vi "template (reverse).vi"() -> ()   [LabVIEW 2012]
uses:
  <vilib>/Analysis/1siggen.llb/Ramp Pattern by Samples.vi
  <vilib>/Analysis/NI_AALBase.lvlib
panel:
  out "Sorted Array":variant[](array[variant])
  out "Sorted Keys":dbl[](array[numeric])
  in  "Keys":dbl[](array[numeric])
  in  "Array":variant[](array[variant])
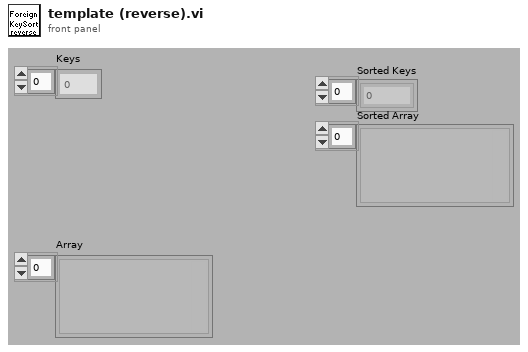
[diagram p1: front panel]
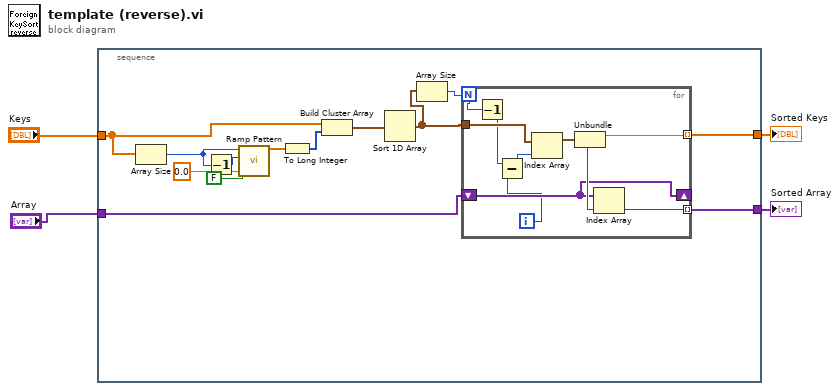
[diagram p0: block diagram]
diagram:
  n1 = stacked-sequence {
    tunnel: "Keys" -> [w11]
    tunnel: "Array" -> [w9]
    tunnel: [w8] -> w2
    tunnel: [w7] -> w1
    frame #0 {
      n2 = Array Size(array=w11) -> (size(s)=w16:i32)
      n3 = Decrement(x=w16) -> (x-1=w17:i32)
      n4 = call-poly <vilib>:"Ramp Pattern.vi"("exclude end?"=FALSE, "start"=0.0, "end"=w17, "samples"=w16) -> ("Ramp Pattern"=w13:dbl[])  [unwired: 6 in, 1 out]
      n5 = To Long Integer(number=w13) -> (32bit integer=w12:i32[])
      n6 = Build Cluster Array(w11, w12) -> (w10:cluster{"Numeric":dbl, i32}[])
      n7 = Sort 1D Array(array=w10) -> (sorted array=w6:cluster{"Numeric":dbl, i32}[])
      n8 = Array Size(array=w6) -> (size(s)=w5:i32)
      n9 = for {
        N: w5 -> [w19]
        tunnel: w6 -> [w27]
        shift-right: [w24] -> _
        shift-left: w9 -> [w24]
        tunnel: [w25] -> w8 mode=indexing
        tunnel: [w23] -> w7 mode=indexing
        i -> [w20]
        n10 = Decrement(x=w19) -> (x-1=w18:i32)
        n11 = Subtract(x=w18, y=w20) -> (x-y=w21:i32)
        n12 = Index Array(array=w27, index=w21) -> (element=w22:cluster{"Numeric":dbl, i32})
        n13 = Unbundle(w22) -> ("Numeric"=w25:dbl, w26:i32)
        n14 = Index Array(array=w24, index=w26) -> (element=w23:variant)
      }
    }
  }
  "Sorted Keys" <- w2
  "Sorted Array" <- w1
